vi "Reset-processed.vi"(8 "error in (no error)":errorcluster, 11 "Object ref in":T1) -> (0 "error out":errorcluster, 3 "Object ref out":T1)   [LabVIEW 2013, in "HardwareCharacterization.lvlib" / "HC-Main.lvclass"]
uses:
  HC-Main.lvclass
  Object-reference.ctl
  HC-Main.lvclass/HC-Main.ctl
  Write Scan file parsed_.vi
  Write Positions converted_.vi
  Write Laser power timed_.vi
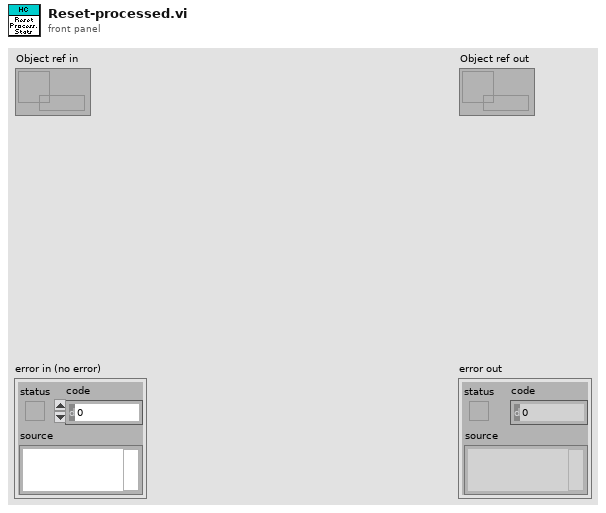
[diagram p1: front panel]
types:
  T1 = typedef "HardwareCharacterization.lvlib/HC-Main.lvclass/Object-reference.ctl" = refnum<data-value>
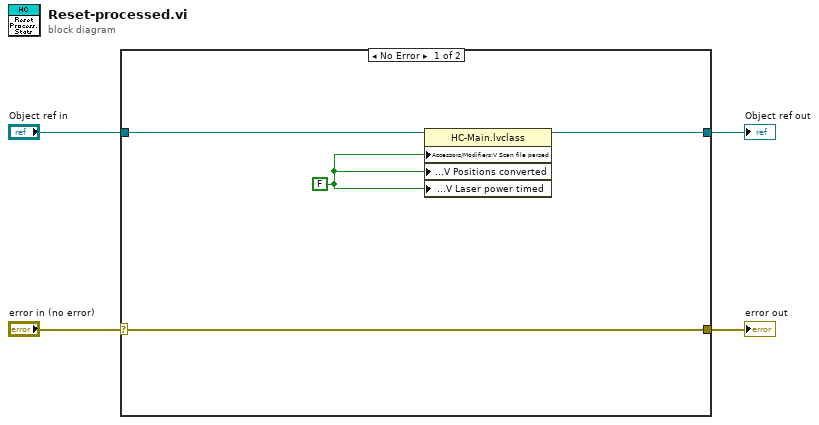
[diagram p0: block diagram]
diagram:
  n1 = case shown="No Error" "error in (no error)" {
    selector: "error in (no error)" -> [w8 w10]
    tunnel: [w8 w10] -> w3
    tunnel: [w6 w9] -> w1
    tunnel: "Object ref in" -> [w7 w9]
    frame No Error {
      w5 = FALSE
      n2 = property class="HC-Main.lvclass"(reference=w7, "Accessors/Modifiers:V Scan file parsed"=w5, "Accessors/Modifiers:V Positions converted"=w5, "Accessors/Modifiers:V Laser power timed"=w5) -> (reference out=w6:T1)  [unwired: 1 in, 1 out]
    }
    frame Error {
    }
  }
  "error out" <- w3
  "Object ref out" <- w1
